vi "Get Request Type.vi"(8 "error in (no error)":errorcluster, 11 "GetSceneItemEnabled in":refnum<class "GetSceneItemEnabled.lvclass">) -> (0 "error out":errorcluster, 2 "Request Type":string, 3 "GetSceneItemEnabled out":refnum<class "GetSceneItemEnabled.lvclass">)   [LabVIEW 2022 SP3, in "obs-websocket-lv.lvlib" / "GetSceneItemEnabled.lvclass"]
uses:
  GetSceneItemEnabled.lvclass
  GetSceneItemEnabled.lvclass/GetSceneItemEnabled.ctl
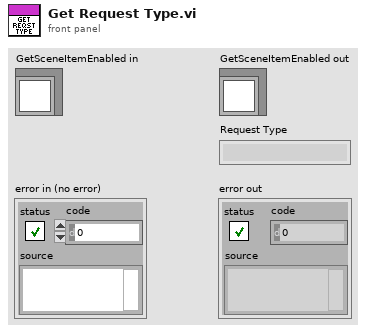
[diagram p1: front panel]
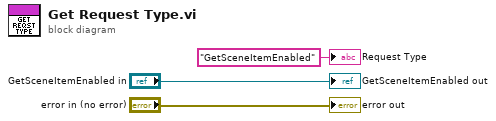
[diagram p0: block diagram]
diagram:
  "error out" <- "error in (no error)"
  "GetSceneItemEnabled out" <- "GetSceneItemEnabled in"
  "Request Type" <- "GetSceneItemEnabled" ("Request Type")
